vi "Report.vi"(8 "error in (no error)":errorcluster, 9 "Received":path, 10 "Approved":path, 11 "Reporter in":refnum<class "Reporter.lvclass">) -> (0 "error out":errorcluster, 3 "Reporter out":refnum<class "Reporter.lvclass">)   [LabVIEW 2020, in "Approval Tests.lvlib" / "Reporter.lvclass"]
uses:
  Reporter.lvclass
  Beyond Compare/Beyond Compare.lvclass
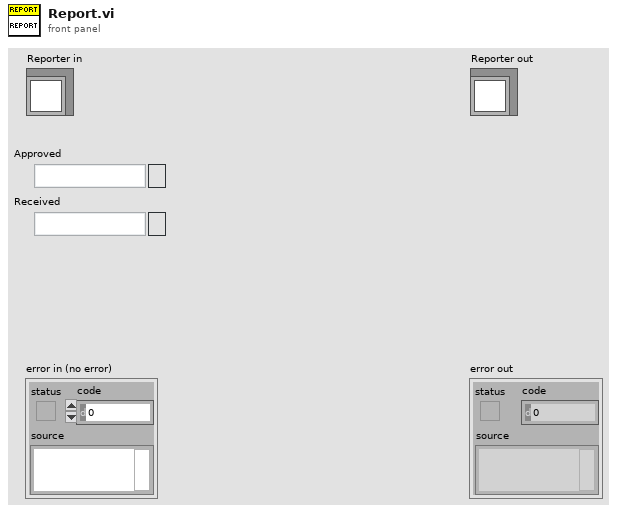
[diagram p1: front panel]
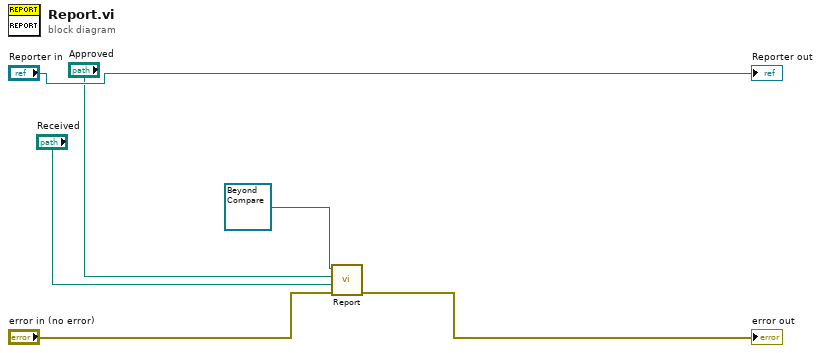
[diagram p0: block diagram]
diagram:
  n1 = call-dynamic "Report.vi"("error in (no error)"="error in (no error)", "Received"="Received", "Approved"="Approved", "Beyond Compare in"=refnum<class "Beyond Compare.lvclass"> refnum ("Approval Tests.lvlib:Beyond Compare.lvclass")) -> ("error out"=→"error out":errorcluster)  [unwired: 6 in, 1 out]
  "Reporter out" <- "Reporter in"
